vi "turn_off_projector.vi"(8 "error in":errorcluster) -> (0 "error out":errorcluster)   [LabVIEW 2019]
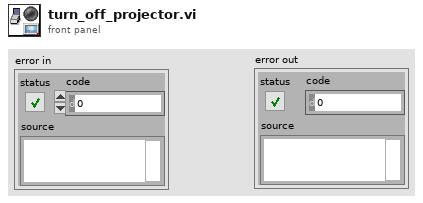
[diagram p1: front panel]
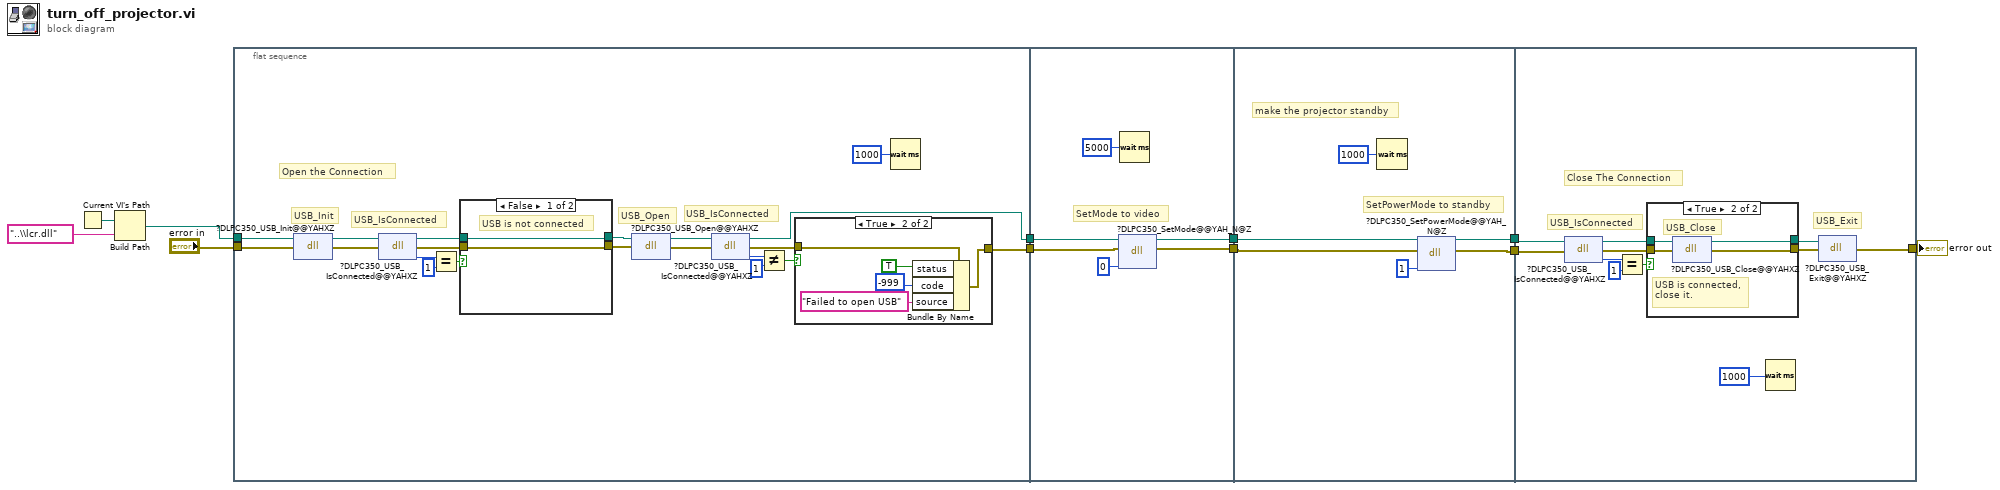
[diagram p0: block diagram]
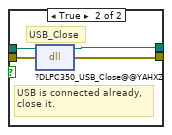
[diagram p3: hidden frame]
diagram:
  n1 = Current VI's Path() -> (path=w8:path)
  n2 = Build Path(base path=w8, name or relative path="..\\lcr.dll") -> (appended path=w6:path)
  n3 = flat-sequence {
    tunnel: [w21] -> w4
    tunnel: "error in" -> [w20]
    tunnel: w6 -> [w19]
    tunnel: [w14] -> w2
    tunnel: w4 -> [w48]
    tunnel: [w47] -> w3
    tunnel: w2 -> [w46]
    tunnel: [w45] -> w1
    tunnel: w3 -> [w52]
    tunnel: [w55] -> w10
    tunnel: w1 -> [w53]
    tunnel: [w54] -> w5
    tunnel: [w61] -> w11
    tunnel: w5 -> [w56]
    tunnel: w10 -> [w57]
    frame #0 {
      # "Open the Connection"
      # "USB_IsConnected"
      # "USB_Open"
      # "USB_IsConnected"
      # "USB_Init"
      n4 = dll-call lib="C:/Users/mochil/Dropbox/LeiferShaevitz/Github/ProjectAPI/LabviewVIs/lcr.dll" fn="?DLPC350_USB_Init@@YAHXZ"(path in=w19, error in=w20) -> (path out=w18:path, error out=w31:errorcluster)  [unwired: 2 in]
      n5 = dll-call lib="C:/Users/mochil/Dropbox/LeiferShaevitz/Github/ProjectAPI/LabviewVIs/lcr.dll" fn="?DLPC350_USB_IsConnected@@YAHXZ"(path in=w18, error in=w31) -> (path out=w17:path, error out=w28:errorcluster, "return type"=w23:i32)  [unwired: 1 in]
      n6 = Equal?(x=w23, y=1) -> (x = y?=w29:bool)
      n7 = case shown="False" w29 {
        tunnel: w28 -> [w39 w43]
        tunnel: [w39 w42] -> w30
        tunnel: w17 -> [w38 w41]
        tunnel: [w38 w40] -> w16
        frame False {
          # "USB is not connected"
        }
        frame True {
          # "USB_Close"
          # "USB is connected already,\nclose it."
          n8 = dll-call lib="C:/Users/mochil/Dropbox/LeiferShaevitz/Github/ProjectAPI/LabviewVIs/lcr.dll" fn="?DLPC350_USB_Close@@YAHXZ"(path in=w41, error in=w43) -> (path out=w40:path, error out=w42:errorcluster)  [unwired: 2 in]
        }
      }
      n9 = dll-call lib="C:/Users/mochil/Dropbox/LeiferShaevitz/Github/ProjectAPI/LabviewVIs/lcr.dll" fn="?DLPC350_USB_Open@@YAHXZ"(path in=w16, error in=w30) -> (path out=w15:path, error out=w27:errorcluster)  [unwired: 2 in]
      n10 = dll-call lib="C:/Users/mochil/Dropbox/LeiferShaevitz/Github/ProjectAPI/LabviewVIs/lcr.dll" fn="?DLPC350_USB_IsConnected@@YAHXZ"(path in=w15, error in=w27) -> (path out=w14:path, error out=w24:errorcluster, "return type"=w13:i32)  [unwired: 1 in]
      n11 = Not Equal?(x=w13, y=1) -> (x != y?=w25:bool)
      n12 = case shown="True" w25 {
        tunnel: w24 -> [w32 w34]
        tunnel: [w32 w33] -> w21
        frame False {
        }
        frame True {
          n13 = Bundle By Name(cluster=w34, "status"=TRUE, "code"=-999, "source"="Failed to open USB") -> (w33:errorcluster)
        }
      }
      n14 = Wait (ms)(milliseconds to wait=u32 1000) -> ()  [unwired: 1 out]
    }
    frame #1 {
      # "SetMode to video"
      n15 = dll-call lib="C:/Users/mochil/Dropbox/LeiferShaevitz/Github/ProjectAPI/LabviewVIs/lcr.dll" fn="?DLPC350_SetMode@@YAH_N@Z"(path in=w46, error in=w48, "SLmode"=0) -> (path out=w45:path, error out=w47:errorcluster)  [unwired: 3 in]
      n16 = Wait (ms)(milliseconds to wait=u32 5000) -> ()  [unwired: 1 out]
    }
    frame #2 {
      # "SetPowerMode to standby"
      # "make the projector standby"
      n17 = Wait (ms)(milliseconds to wait=u32 1000) -> ()  [unwired: 1 out]
      n18 = dll-call lib="C:/Users/mochil/Dropbox/LeiferShaevitz/Github/ProjectAPI/LabviewVIs/lcr.dll" fn="?DLPC350_SetPowerMode@@YAH_N@Z"(path in=w53, error in=w52, "Standby"=1) -> (path out=w54:path, error out=w55:errorcluster)  [unwired: 3 in]
    }
    frame #3 {
      # "Close The Connection"
      # "USB_Exit"
      # "USB_IsConnected"
      n19 = dll-call lib="C:/Users/mochil/Dropbox/LeiferShaevitz/Github/ProjectAPI/LabviewVIs/lcr.dll" fn="?DLPC350_USB_IsConnected@@YAHXZ"(path in=w56, error in=w57) -> (path out=w60:path, error out=w64:errorcluster, "return type"=w65:i32)  [unwired: 1 in]
      n20 = Equal?(x=w65, y=1) -> (x = y?=w63:bool)
      n21 = case shown="True" w63 {
        tunnel: w64 -> [w68 w72]
        tunnel: [w68 w71] -> w66
        tunnel: w60 -> [w67 w70]
        tunnel: [w67 w69] -> w59
        frame False {
          # "USB is not connected"
        }
        frame True {
          # "USB_Close"
          # "USB is connected,\nclose it."
          n22 = dll-call lib="C:/Users/mochil/Dropbox/LeiferShaevitz/Github/ProjectAPI/LabviewVIs/lcr.dll" fn="?DLPC350_USB_Close@@YAHXZ"(path in=w70, error in=w72) -> (path out=w69:path, error out=w71:errorcluster)  [unwired: 2 in]
        }
      }
      n23 = Wait (ms)(milliseconds to wait=u32 1000) -> ()  [unwired: 1 out]
      n24 = dll-call lib="C:/Users/mochil/Dropbox/LeiferShaevitz/Github/ProjectAPI/LabviewVIs/lcr.dll" fn="?DLPC350_USB_Exit@@YAHXZ"(path in=w59, error in=w66) -> (error out=w61:errorcluster)  [unwired: 2 in, 1 out]
    }
  }
  "error out" <- w11
